vi "array sales ex 3.vi"() -> ()   [LabVIEW 2020]
panel:
  out "size(s)":i32[](array[numeric])
  out "COLUMN SUM":dbl
  out "subarray 2":string[](array[string])
  out "SEARCH SALES DATA ARRAY":string[][](array[string])
  in  "Search Value":string
  out "subarray":string[](array[string])
  in  "COLUMN HEADING":T1(ring)
  out "sales data":string[][](array[string])
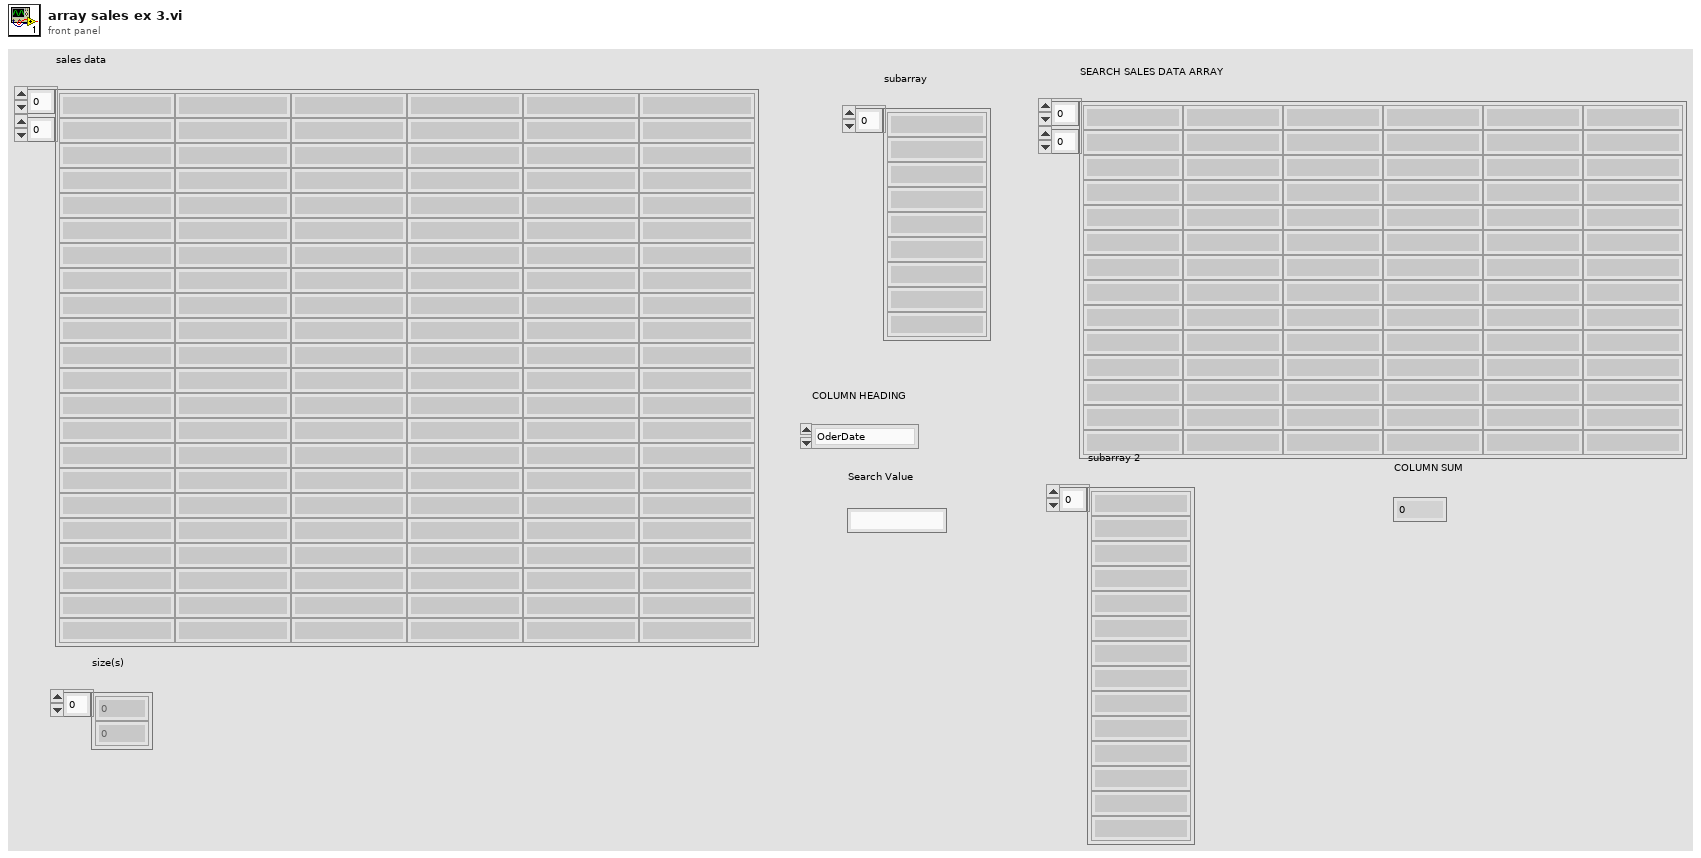
[diagram p1: front panel]
types:
  T1 = enum16{"OderDate", "Region", "Rep", "Item", "Units", "UnitCost"}
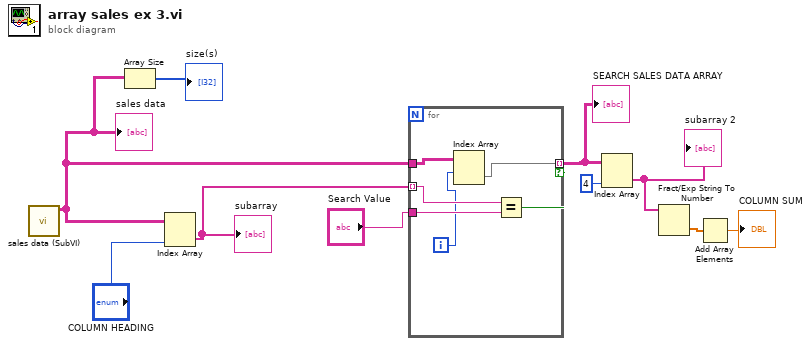
[diagram p0: block diagram]
diagram:
  n1 = call "sales data (SubVI).vi"() -> ("sales data"=w2:string[][])  [unwired: 11 in]
  "sales data" <- w2
  n2 = Array Size(array=w2) -> (size(s)=→"size(s)":i32[])
  n3 = Index Array(array=w2, index (col)="COLUMN HEADING") -> (element=w10:string[])  [unwired: 1 in]
  "subarray" <- w10
  n4 = for {
    tunnel: w10 -> [w14] mode=indexing
    tunnel: "Search Value" -> [w16]
    tunnel: w2 -> [w13]
    tunnel: [w11] -> w8 mode=indexing if=w15
    i -> [w12]
    n5 = Index Array "Index Array"(array=w13, index (row)=w12) -> (element=w11:string[])  [unwired: 1 in]
    n6 = Equal?(x=w14, y=w16) -> (x = y?=w15:bool)
  }
  "SEARCH SALES DATA ARRAY" <- w8
  n7 = Index Array(array=w8, index (col)=4 ("disabled index (col)")) -> (element=w5:string[])  [unwired: 1 in]
  "subarray 2" <- w5
  n8 = Fract/Exp String To Number(string=w5) -> (number=w4:dbl[])  [unwired: 3 in, 1 out]
  n9 = Add Array Elements(numeric array=w4) -> (sum=→"COLUMN SUM":dbl)
